vi "Abort.vi"(8 "error in (no error)":errorcluster, 11 "VISA resource name":refnum<visa-resource-name>) -> (0 "error out":errorcluster, 3 "VISA resource name out":refnum<visa-resource-name>)   [LabVIEW 2020, in "Counter.lvlib" / "PICOTEST U62XXA series.lvlib"]
doc: "Causes the Counter to abort, as quickly as possible, any measurement in progress.\n\n<B>Note:</B>\n\nAborting a measurement in progress <B>invalidates</B> the result, with one <B>exception</B>. Calling the Abort VI is the appropriate way to <B>terminate</B> an <B>Auto Armed (Continuous) totalize measurement</B>. The abort VI has to be called before data is fetched."
uses:
  PICOTEST U62XXA series.lvlib
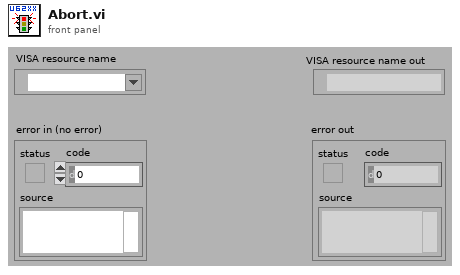
[diagram p1: front panel]
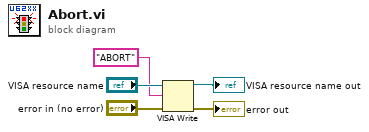
[diagram p0: block diagram]
diagram:
  n1 = VISA Write(VISA resource name="VISA resource name", write buffer="ABORT", error in (no error)="error in (no error)") -> (VISA resource name out=→"VISA resource name out":refnum<visa-resource-name>, error out=→"error out":errorcluster)  [unwired: 1 out]
